vi "Get Filepath.vi"(8 "error in":errorcluster, 11 "FileHandler in":refnum<class "RotateFileHandler.lvclass">) -> (0 "error out":errorcluster, 2 "Filepath":path, 3 "FileHandler out":refnum<class "RotateFileHandler.lvclass">)   [LabVIEW 2024, in "RotateFileHandler.lvclass"]
doc: "____\nHAMPEL SOFTWARE ENGINEERING v2.2.2 (2025-01-16 15:41)"
uses:
  RotateFileHandler.lvclass
  RotateFileHandler.lvclass/RotateFileHandler.ctl
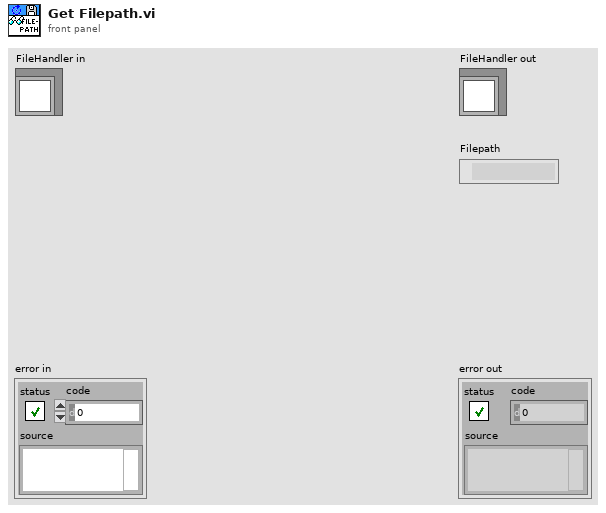
[diagram p1: front panel]
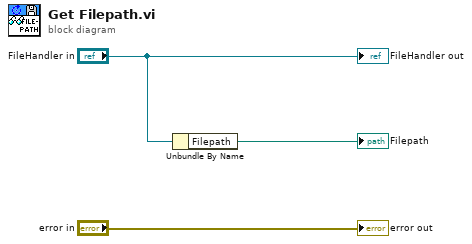
[diagram p0: block diagram]
diagram:
  n1 = Unbundle By Name("FileHandler in") -> ("Filepath"=→"Filepath":path)
  "error out" <- "error in"
  "FileHandler out" <- "FileHandler in"
